vi "Set PluginCore RefreshStatistics Response.vi"(7 "Streaming? (F)":bool, 8 "error in (no error)":errorcluster, 10 "Message Data":T1, 11 "gRPCid in":T2) -> (0 "error out":errorcluster)   [LabVIEW 2021, in "CIF_Plugin_Core_server.lvlib" / "PluginCore.lvclass"]
uses:
  PluginCore.lvclass
  <vilib>/gRPC/LabVIEW gRPC Library/Shared/grpcId.ctl
  PluginCore.lvclass/PluginCore.ctl
  CIF_Plugin_Core_server.lvlib
  <vilib>/gRPC/LabVIEW gRPC Library/grpc-lvsupport-release.lvlib
  RPC Messages/cif_plugincore_Status.ctl
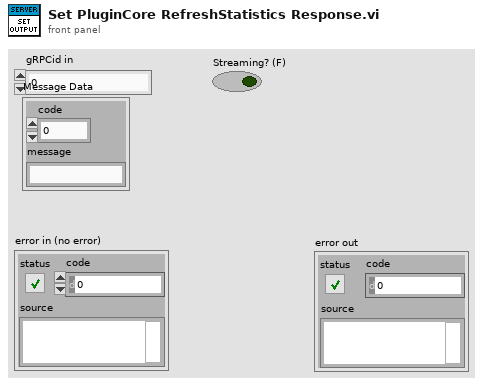
[diagram p1: front panel]
types:
  T1 = typedef "CIF_Plugin_Core_server.lvlib/cif_plugincore_Status.ctl" = cluster{"code":i32, "message":string}
  T2 = typedef "grpc-lvsupport-release.lvlib/grpcId.ctl" = u64
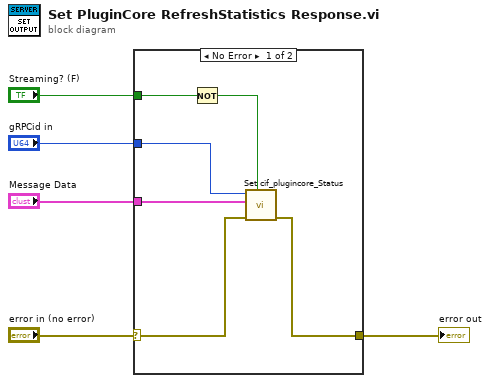
[diagram p0: block diagram]
diagram:
  n1 = case shown="No Error" "error in (no error)" {
    selector: "error in (no error)" -> [w11 w12]
    tunnel: [w9 w12] -> w4
    tunnel: "gRPCid in" -> [w10 _]
    tunnel: "Message Data" -> [w8 _]
    tunnel: "Streaming? (F)" -> [w7 _]
    frame No Error {
      n2 = Not(x=w7) -> (.not. x?=w6:bool)
      n3 = call "Set cif_plugincore_Status.vi"("Complete Call (T)"=w6, "error in (no error)"=w11, "package_templatemessage"=w8, "gRPCid"=w10) -> ("error out"=w9:errorcluster)  [unwired: 7 in]
    }
    frame Error {
    }
  }
  "error out" <- w4
